vi "Change Camera.vi"(0 "Display State In":T1 {"Centroid"."Y Centroid" format="%.2f"; "Centroid"."X Centroid" format="%.2f"; "ROI"."Contours"."Type" items=["No Selection", "Point", "Line", "Rectangle", "Oval", "Polygon", "Freehand Region", "Annulus", "Unused2", "Unused3", "Broken Line", "Freehand Line", "Rotated Rectangle"]}, 5 "IMAQdx Cam":refnum<class "IMAQdx Cam.lvclass">, 9 "Container State":T7, 11 "error in (no error)":errorcluster) -> (4 "Display State Out":T1 {"Centroid"."Y Centroid" format="%.2f"; "Centroid"."X Centroid" format="%.2f"; "ROI"."Contours"."Type" items=["No Selection", "Point", "Line", "Rectangle", "Oval", "Polygon", "Freehand Region", "Annulus", "Unused2", "Unused3", "Broken Line", "Freehand Line", "Rotated Rectangle"]}, 6 "cnfg file old cam":path, 15 "error out":errorcluster)   [LabVIEW 2009, in "POLARIS IMAQ Display.xctl"]
uses:
  POLARIS IMAQ Display.xctl
  <vilib>/_xctls/Container State.ctl
  State.ctl
  IMAQdx Cam/IMAQdx Cam.lvclass
  Properties/ImageSource.ctl
  <vilib>/vision/Image Controls.llb/IMAQ Image.ctl
  DisplaySettings.ctl
  Named ROI.ctl
  Analyze Classes/Analyze BaseClass/Analyze BaseClass.lvclass
  Palette.ctl
  <vilib>/_xctls/XControlSupport.lvlib
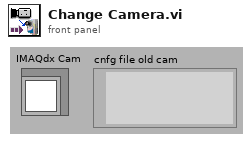
[diagram p1: front panel]
types:
  T1 = typedef "POLARIS IMAQ Display.xctl/State.ctl" = cluster{"ImageSource":T2, "IMAQdx Cam":refnum<class "IMAQdx Cam.lvclass">, "WorkDir":path, "Image Name Prefix":string, "ROI":T3, "BG Image":T4, "Display Image":T4, "Display settings":T5, "Mask image":T4, "ConfigDir":path, "Display ref":refnum<vi>, "Saved ROIs":T6[], "Selected ROI":string, "Analyze Objects":refnum<class "Analyze BaseClass.lvclass">[], "Analysis Params":variant, "Analysis Results":variant, "Overlays?":bool[], "Ref Palette type":refnum<vi>, "Time in Filename?":bool, "Save Report?":bool, "Appl Params":variant, "Show ZoomBtn?":bool, "Image file":path, "SubstractBG?":bool, "Centroid":cluster{"X Centroid":sgl, "Y Centroid":sgl}, "Image In":T4}
  T2 = typedef "POLARIS IMAQ Display.xctl/ImageSource.ctl" = enum16{"Camera", "File"}
  T3 = typedef "ROI Descriptor" = cluster{"Global Rectangle":i32[], "Contours":cluster{"ID":enum32{"External", "Internal"}, "Type":u32, "Coordinates":i32[]}[]}
  T4 = typedef "IMAQ Image.ctl" = refnum<image>
  T5 = typedef "POLARIS IMAQ Display.xctl/DisplaySettings.ctl" = cluster{"Min. Thresh.":sgl, "X":dbl, "Y":dbl, "ShowLineout":bool, "ScaleParts":i32, "ShowLegende":bool, "Target Cross":bool, "Centroid Cross":bool, "Target color":u32, "Centroid color":u32, "calibr. mm/px":sgl}
  T6 = typedef "POLARIS IMAQ Display.xctl/Named ROI.ctl" = cluster{"ROI":cluster{"Global Rectangle":i32[], "Contours":cluster{"Contour Type":u32, "ROI Type":u32, "Points":i32[]}[]}, "Name":string}
  T7 = typedef "XControlSupport.lvlib/Container State.ctl" = cluster{"Indicator?":bool, "Run Mode?":bool, " Refnum":refnum<vi>}
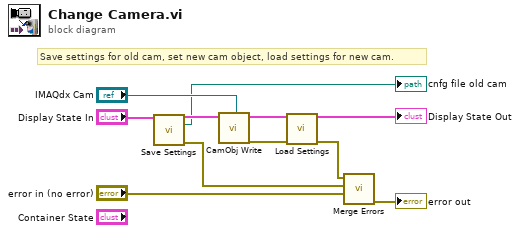
[diagram p0: block diagram]
diagram:
  # "Save settings for old cam, set new cam object, load settings for new cam."
  n1 = call "Save Settings.vi"("Display State In"="Display State In") -> ("Display State Out"=w10:T1, "file path out"=→"cnfg file old cam":path, "error out"=w3:errorcluster)  [unwired: 12 in]
  n2 = call "CamObj Write.vi"("Value"="IMAQdx Cam", "Display State In"=w10) -> ("error out"=w6:errorcluster, "Display State Out"=w8:T1)  [unwired: 4 in]
  n3 = call "Load Settings.vi"("Display State In"=w8, "error in (no error)"=w6) -> ("Display State Out"=→"Display State Out":T1, "error out"=w4:errorcluster)  [unwired: 12 in]
  n4 = call <vilib>:"Merge Errors.vi"("error in 3 (no error)"="error in (no error)", "error in 2 (no error)"=w3, "error in 1 (no error)"=w4) -> ("error out"=→"error out":errorcluster)  [unwired: 4 in]
